vi "Untitled 3.vi"() -> ()   [LabVIEW 2018]
uses:
  <vilib>/Utility/miscctls.llb/LVStringsAndValuesArrayTypeDef_U16.ctl
panel:
  out "Value":u16
  out "Ring Text.Text":string
  in  "Strings And Values [] 2":T1
  out "Strings And Values []":T1
  in  "Ring 3":u16(ring) items=["A"=1, "B"=3, "C"=5, "D"=7]
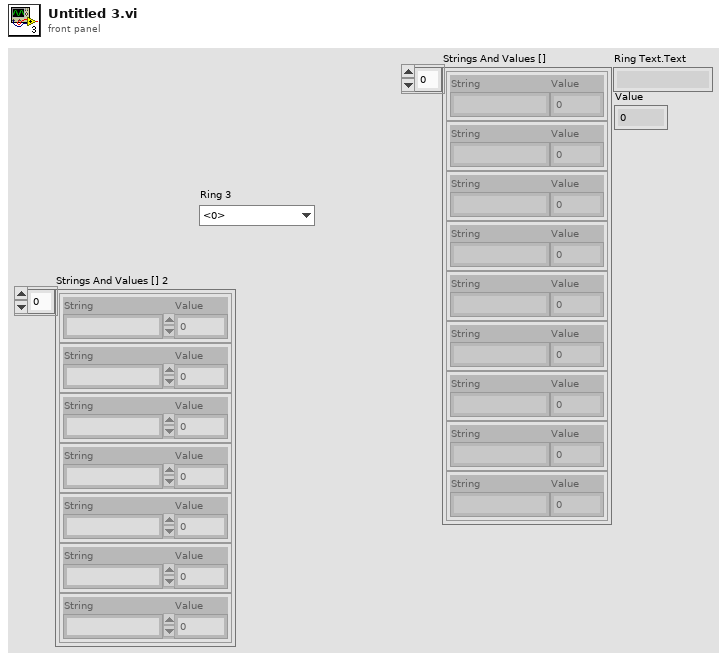
[diagram p1: front panel]
types:
  T1 = typedef "LVStringsAndValuesArrayTypeDef_U16.ctl" = cluster{"String":string, "Value":u16}[]
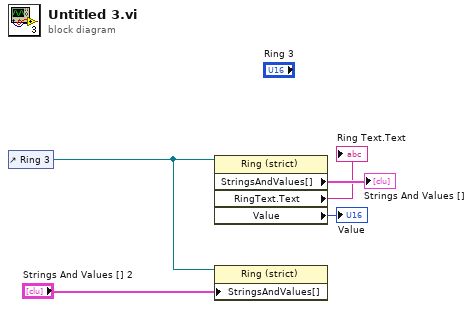
[diagram p0: block diagram]
diagram:
  n1 = control-ref of="Ring 3"() -> (w4:refnum<vi>)
  n2 = property class="Ring (strict)"(reference=w4) -> ("StringsAndValues[]"=→"Strings And Values []":T1, "RingText.Text"=→"Ring Text.Text":string, "Value"=→"Value":u16)  [unwired: 1 in, 2 out]
  n3 = property class="Ring (strict)"(reference=w4, "StringsAndValues[]"="Strings And Values [] 2") -> ()  [unwired: 1 in, 2 out]
